vi "QMH_Enqueue RR.vi"(6 "Reply":T1, 7 "Priority Message? (F)":bool, 8 "error in":errorcluster, 9 "Message Data":variant, 10 "Message":string, 11 "Message Queue in":refnum<class "ModuleQueue.lvclass">) -> (0 "error out":errorcluster, 3 "Message Queue out":refnum<class "ModuleQueue.lvclass">)   [LabVIEW 2024, in "ModuleShared.lvlib"]
doc: "For a regular message, enqueue the message. For a priority message, enqueue it at the front of the queue.\nThis is an instance of the polymorphic VI: \"Enqueue Message (poly).vi\"\n____\nDQMH Framework: Palette 7.1.0.1503\nCopyright (c) 2025, DQMH Consortium"
uses:
  Shared/ModuleShared.lvlib
  ModuleQueue.lvclass
  ModuleCore/Reply.ctl
  ModuleQueue.lvclass/ModuleQueue.ctl
  ModuleCore/Module.lvclass
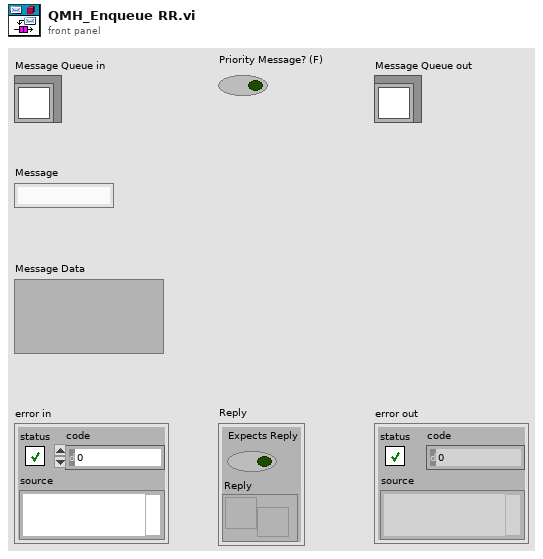
[diagram p1: front panel]
types:
  T1 = typedef "Module.lvclass/Reply.ctl" = cluster{"Expects Reply":bool, "Reply":refnum<notifier>}
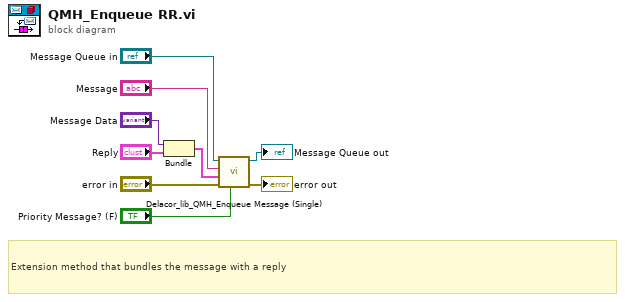
[diagram p0: block diagram]
diagram:
  # "Extension method that bundles the message with a reply"
  n1 = Bundle("Message Data"="Message Data", "Reply"="Reply") -> (w2:cluster{"Message Data":variant, "Reply":T1})  [unwired: 1 in]
  n2 = call "Delacor_lib_QMH_Enqueue Message (Single).vi"("Priority Message? (F)"="Priority Message? (F)", "error in"="error in", "Message Data"=w2, "Message"="Message", "Message Queue in"="Message Queue in") -> ("error out"=→"error out":errorcluster, "Message Queue out"=→"Message Queue out":refnum<class "ModuleQueue.lvclass">)  [unwired: 5 in]
